vi "Bertta_v09_8.vi"() -> ()   [LabVIEW 2015]
panel:
  out "element":bool
  out "Started:":string
  in  "SHUTDOWN":bool
  in  "MASTER CONTROL":bool
  in  "Tab Control":T1(tab)
  in  "Read Seq":bool
  in  "Save Seq":bool
  in  "Configuration file":path=path "C:/Users/shresplab/Desktop/BerttaConfiguration.lvm" caption="Filename"
  in  "OK Button 2":bool
  out "Boolean":bool
  in  "User (initials)":string
  in  "Project name":string
  in  "Description":string
  out "Output file":string
  out "PUMP1":bool
  out "Target amount":dbl
  out "Scale weight":dbl
  out "Amount now":dbl
  out "Flow rate":dbl
  out "Time to target":dbl format="%<%H:%M:%S>t"
  out "Current step":dbl
  out "Target":dbl
  out "Amount now":dbl
  out "Amount now":dbl
  out "Target":dbl
  out "Current step":dbl
  out "Time to target":dbl format="%<%H:%M:%S>t"
  out "Flow rate":dbl
  out "Amount now":dbl
  out "Scale weight":dbl
  out "Target amount":dbl
  out "PUMP2":bool
  out "Sensor OK 6":bool
  out "Sensor OK 5":bool
  out "Sensor OK 4":bool
  out "Sensor OK 3":bool
  in  "OK Button":bool
  in  "Add comment":string
  out "PUMP3":bool
  out "Target amount":dbl
  out "Scale weight":dbl
  out "Amount now":dbl
  out "Flow rate":dbl
  out "Time to target":dbl format="%<%H:%M:%S>t"
  out "Current step":dbl
  out "Target":dbl
  out "Amount now":dbl
  out "Tr":dbl
  out "Tj in":dbl
  out "Tj out":dbl
  out "T set":dbl
  out "Current step":i32
  out "RPM":dbl
  out "Torque 2":dbl
  out "Waveform Chart 5":dynamicdata(graph)
  out "Waveform Chart 6":dynamicdata(graph)
  out "Waveform Chart 7":dynamicdata(graph)
  in  "Tab Control 2":T2(tab)
  out "Waveform Chart 3":dynamicdata(graph)
  out "Waveform Chart 8":dynamicdata(graph)
  out "Waveform Chart 11":dynamicdata(graph)
  out "Waveform Chart 13":dynamicdata(graph)
  out "Waveform Chart 9":dynamicdata(graph)
  out "Table":string[][](table)=[["14.8.2017 18.06.59", "0,000000", "417,670000", "-0,150000", "1,000000", "22,220000", "23,366837", "23,574959", "23,985852", "23,690000", "240,000000", "4,000000", "0,000000", "397,000000", "-397,000000", "1,000000"], ["14.8.2017 18.07.06", "0,000000", "417,640000", "-0,120000", "1,000000", "22,220000", "23,763115", "23,906257", "23,985694", "23,680000", "240,000000", "4,000000", "0,000000", "397,000000", "-397,000000", "1,000000"], ["14.8.2017 18.07.13", "0,000000", "417,640000", "-0,120000", "1,000000", "22,220000", "23,965922", "24,013440", "23,984906", "23,670000", "240,000000", "4,100000", "3,000000", "397,000000", "-397,000000", "1,000000"], ["14.8.2017 18.07.21", "0,000000", "417,640000", "-0,120000", "1,000000", "22,220000", "23,943860", "23,900110", "23,987113", "23,670000", "240,000000", "4,000000", "0,000000", "397,000000", "-397,000000", "1,000000"], ["14.8.2017 18.07.28", "0,000000", "417,640000", "-0,120000", "1,000000", "22,220000", "23,736328", "23,600018", "23,989004", "23,660000", "240,000000", "4,000000", "0,000000", "397,000000", "-397,000000", "1,000000"], ["14.8.2017 18.07.36", "0,000000", "417,640000", "-0,120000", "1,000000", "22,220000", "23,480910", "23,324538", "23,991053", "23,660000", "240,000000", "4,000000", "0,000000", "397,000000", "-397,000000", "1,000000"], ["14.8.2017 18.07.43", "0,000000", "417,640000", "-0,120000", "2,000000", "22,220000", "23,195579", "23,008270", "23,999093", "23,650000", "240,000000", "4,000000", "0,000000", "397,000000", "-397,000000", "1,000000"], ["14.8.2017 18.07.51", "0,000000", "417,650000", "-417,650000", "1,000000", "22,220000", "22,862541", "22,649021", "24,003979", "23,650000", "240,000000", "4,000000", "0,000000", "397,000000", "-397,000000", "2,000000"], ["14.8.2017 18.07.58", "0,000000", "417,640000", "0,010000", "1,000000", "22,220000", "22,541353", "22,354878", "24,005398", "23,650000", "240,000000", "4,000000", "0,000000", "397,000000", "-397,000000", "1,000000"], ["14.8.2017 18.08.06", "0,000000", "417,640000", "0,010000", "1,000000", "22,220000", "22,347931", "22,253738", "24,007605", "23,640000", "240,000000", "4,100000", "0,000000", "397,000000", "-397,000000", "1,000000"], ["14.8.2017 18.08.13", "0,000000", "417,640000", "0,010000", "1,000000", "22,220000", "22,329030", "22,302102", "24,006028", "23,640000", "240,000000", "4,000000", "0,000000", "395,820000", "-395,820000", "1,000000"], ["14.8.2017 18.08.20", "0,000000", "417,640000", "0,010000", "1,000000", "22,220000", "22,466849", "22,511320", "24,002403", "23,630000", "240,000000", "4,000000", "0,000000", "395,830000", "-0,010000", "1,000000"], ["14.8.2017 18.08.28", "0,000000", "417,640000", "0,010000", "1,000000", "22,220000", "22,707062", "22,835101", "24,000984", "23,620000", "240,000000", "4,000000", "0,000000", "395,830000", "-0,010000", "1,000000"], ["14.8.2017 18.08.35", "0,000000", "417,640000", "0,010000", "1,000000", "22,220000", "23,054104", "23,232979", "24,001299", "23,600000", "240,000000", "4,000000", "0,000000", "395,830000", "-0,010000", "1,000000"], ["14.8.2017 18.08.43", "0,000000", "417,640000", "0,010000", "1,000000", "22,220000", "23,412371", "23,522793", "24,002560", "23,590000", "240,000000", "4,000000", "0,000000", "395,820000", "0,000000", "1,000000"], ["14.8.2017 18.08.51", "0,000000", "417,640000", "0,010000", "1,000000", "22,220000", "23,596247", "23,656125", "24,003821", "23,580000", "240,000000", "4,000000", "0,000000", "395,820000", "0,000000", "1,000000"]]
  in  "Reset":bool
  in  "Temp5":dbl=20.0
  in  "Temp4":dbl=30.0
  in  "Temp3":dbl=40.0
  in  "Temp2":dbl=30.0
  in  "Temp1":dbl=20.0
  out "Boolean 12":bool
  out "Boolean 7":bool
  out "Boolean 6":bool
  out "Boolean 5":bool
  out "Boolean 4":bool
  out "Boolean 19":bool
  in  "Time1":dbl=5.0
  in  "Time2":dbl=5.0
  in  "Time3":dbl=5.0
  in  "Time4":dbl=5.0
  in  "T ext / T ext 2":enum32{"External 1", "External 2"}(radio)
  out "Sensor OK":bool
  in  "T fail":dbl=20.0
  in  "?":bool
  in  "T manual setpoint":dbl=20.0
  in  "Lauda port":dbl=9.0
  in  "Manual select":enum32{"Tr", "Tj"}(radio)
  in  "PAUSE":bool
  out "Waveform Chart":dynamicdata(graph)
  out "T external 2":dbl
  out "Led11 5":bool
  in  "Radio Buttons 4":enum32{"Reglo Digital", "Reglo Analog", "PAM"}(radio)
  out "Speed":dbl
  out "mA":dbl format="%#_2g"
  in  "Port":i32=16
  out "RPM":dbl format="%_4f"
  out "Led10 3":bool
  out "Led9 3":bool
  out "Led8 3":bool
  out "Led7 3":bool
  out "Led6 3":bool
  out "Led5 3":bool
  out "Led4 3":bool
  out "Led3 3":bool
  out "Led2 3":bool
  out "Led1 3":bool
  in  "PumpSeq 4":dbl[][](array[numeric])=[[1.0, 1.0, 0.0, 0.0, 0.0, 0.0, 0.0, 0.0, 0.0, 0.0], [2.0, 1.0, 0.0, 0.0, 0.0, 0.0, 0.0, 0.0, 0.0, 0.0], [3.0, 1.0, 0.0, 0.0, 0.0, 0.0, 0.0, 0.0, 0.0, 0.0], [0.0, 0.0, 0.0, 0.0, 0.0, 0.0, 0.0, 0.0, 0.0, 0.0], [0.0, 0.0, 0.0, 0.0, 0.0, 0.0, 0.0, 0.0, 0.0, 0.0], [0.0, 0.0, 0.0, 0.0, 0.0, 0.0, 0.0, 0.0, 0.0, 0.0], [0.0, 0.0, 0.0, 0.0, 0.0, 0.0, 0.0, 0.0, 0.0, 0.0], [0.0, 0.0, 0.0, 0.0, 0.0, 0.0, 0.0, 0.0, 0.0, 0.0], [0.0, 0.0, 0.0, 0.0, 0.0, 0.0, 0.0, 0.0, 0.0, 0.0], [0.0, 0.0, 0.0, 0.0, 0.0, 0.0, 0.0, 0.0, 0.0, 0.0]]
  in  "?":bool
  out "Flow rate (g/min)":dbl
  out "Scale reading":dbl
  out "Step amount now":dbl
  in  "Grams / min":dbl
  out "Waveform Chart 14":dynamicdata(graph)
  in  "?":bool
  out "Total amount now":dbl
  out "Led11 4":bool
  in  "Reset 5":bool
  out "Elapsed / step":i32
  out "Time to target":dbl format="%<%H:%M:%S>t"
  out "Led11":bool
  in  "Radio Buttons 2":enum32{"Reglo Digital", "Reglo Analog", "PAM"}(radio)
  out "Speed":dbl
  out "mA":dbl format="%#_2g"
  in  "Port":i32=15
  out "RPM":dbl format="%_4f"
  out "Led10":bool
  out "Led9":bool
  out "Led8":bool
  out "Led7":bool
  out "Led6":bool
  out "Led5":bool
  out "Led4":bool
  out "Led3":bool
  out "Led2":bool
  out "Led1":bool
  in  "PumpSeq 2":dbl[][](array[numeric])=[[0.0, 0.0, 0.0, 0.0, 0.0, 0.0, 0.0, 0.0, 0.0, 0.0], [0.0, 0.0, 0.0, 0.0, 0.0, 0.0, 0.0, 0.0, 0.0, 0.0], [0.0, 0.0, 0.0, 0.0, 0.0, 0.0, 0.0, 0.0, 0.0, 0.0], [0.0, 0.0, 0.0, 0.0, 0.0, 0.0, 0.0, 0.0, 0.0, 0.0], [0.0, 0.0, 0.0, 0.0, 0.0, 0.0, 0.0, 0.0, 0.0, 0.0], [0.0, 0.0, 0.0, 0.0, 0.0, 0.0, 0.0, 0.0, 0.0, 0.0], [0.0, 0.0, 0.0, 0.0, 0.0, 0.0, 0.0, 0.0, 0.0, 0.0], [0.0, 0.0, 0.0, 0.0, 0.0, 0.0, 0.0, 0.0, 0.0, 0.0], [0.0, 0.0, 0.0, 0.0, 0.0, 0.0, 0.0, 0.0, 0.0, 0.0], [0.0, 0.0, 0.0, 0.0, 0.0, 0.0, 0.0, 0.0, 0.0, 0.0]]
  in  "?":bool
  out "Flow rate (g/min)":dbl
  out "Scale reading":dbl
  out "Step amount now":dbl
  in  "Grams / min":dbl
  out "Waveform Chart 10":dynamicdata(graph)
  in  "?":bool
  out "Total amount now":dbl
  out "Led11":bool
  in  "Reset 3":bool
  out "Elapsed / step":i32
  out "Time to target":dbl format="%<%H:%M:%S>t"
  out "Led11 3":bool
  in  "Radio Buttons 3":enum32{"Reglo Digital", "Reglo Analog", "PAM"}(radio)
  out "Speed":dbl
  out "mA":dbl format="%#_2g"
  in  "Port":i32=14
  out "RPM":dbl format="%_4f"
  out "Led10 2":bool
  out "Led9 2":bool
  out "Led8 2":bool
  out "Led7 2":bool
  out "Led6 2":bool
  out "Led5 2":bool
  out "Led4 2":bool
  out "Led3 2":bool
  out "Led2 2":bool
  out "Led1 2":bool
  in  "PumpSeq 3":dbl[][](array[numeric])=[[1.0, 3.0, 0.0, 0.0, 0.0, 0.0, 0.0, 0.0, 0.0, 0.0], [2.0, 3.0, 0.0, 0.0, 0.0, 0.0, 0.0, 0.0, 0.0, 0.0], [3.0, 3.0, 0.0, 0.0, 0.0, 0.0, 0.0, 0.0, 0.0, 0.0], [0.0, 0.0, 0.0, 0.0, 0.0, 0.0, 0.0, 0.0, 0.0, 0.0], [0.0, 0.0, 0.0, 0.0, 0.0, 0.0, 0.0, 0.0, 0.0, 0.0], [0.0, 0.0, 0.0, 0.0, 0.0, 0.0, 0.0, 0.0, 0.0, 0.0], [0.0, 0.0, 0.0, 0.0, 0.0, 0.0, 0.0, 0.0, 0.0, 0.0], [0.0, 0.0, 0.0, 0.0, 0.0, 0.0, 0.0, 0.0, 0.0, 0.0], [0.0, 0.0, 0.0, 0.0, 0.0, 0.0, 0.0, 0.0, 0.0, 0.0], [0.0, 0.0, 0.0, 0.0, 0.0, 0.0, 0.0, 0.0, 0.0, 0.0]]
  in  "?":bool
  out "Flow rate (g/min)":dbl
  out "Scale reading":dbl
  out "Step amount now":dbl
  in  "Grams / min":dbl
  out "Waveform Chart 12":dynamicdata(graph)
  in  "?":bool
  out "Total amount now":dbl
  out "Led11 2":bool
  in  "Reset 4":bool
  out "Elapsed / step":i32
  out "Time to target":dbl format="%<%H:%M:%S>t"
  in  "Bypass select 2":enum32{"Remote", "Manual"}(radio)=enum."Manual"
  in  "Port":dbl=13.0
  out "RPM":dbl
  out "Torque":dbl
  in  "Set RPM":dbl(slide) scale=0.0..2000.0
  out "Waveform Chart 4":dynamicdata(graph)
  in  "Treshold (T/C)":dbl=0.5
  out "DAQ 9217 (PT100)":errorcluster
  out "Config File":dbl[][](array[numeric])
  # "Temperature sensor:"
  # "Manual control:"
  # "PUMP & SCALE 1"
  # "STEP"
  # "TOTAL"
  # "PUMP & SCALE 2"
  # "STEP"
  # "TOTAL"
  # "PUMP & SCALE 3"
  # "STEP"
  # "TOTAL"
  # "Manual control"
  # "Secondary temperature sensor"
  # "Device communication"
  # "Temp"
  # "Time"
  # "Grams    /   min"
  # "End of sequence"
  # "Manual control"
  # "Device communication"
  # "Pump configuration"
  # "Grams    /   min"
  # "End of sequence"
  # "Manual control"
  # "Device communication"
  # "Pump configuration"
  # "Grams    /   min"
  # "End of sequence"
  # "Manual control"
  # "Device communication"
  # "Pump configuration"
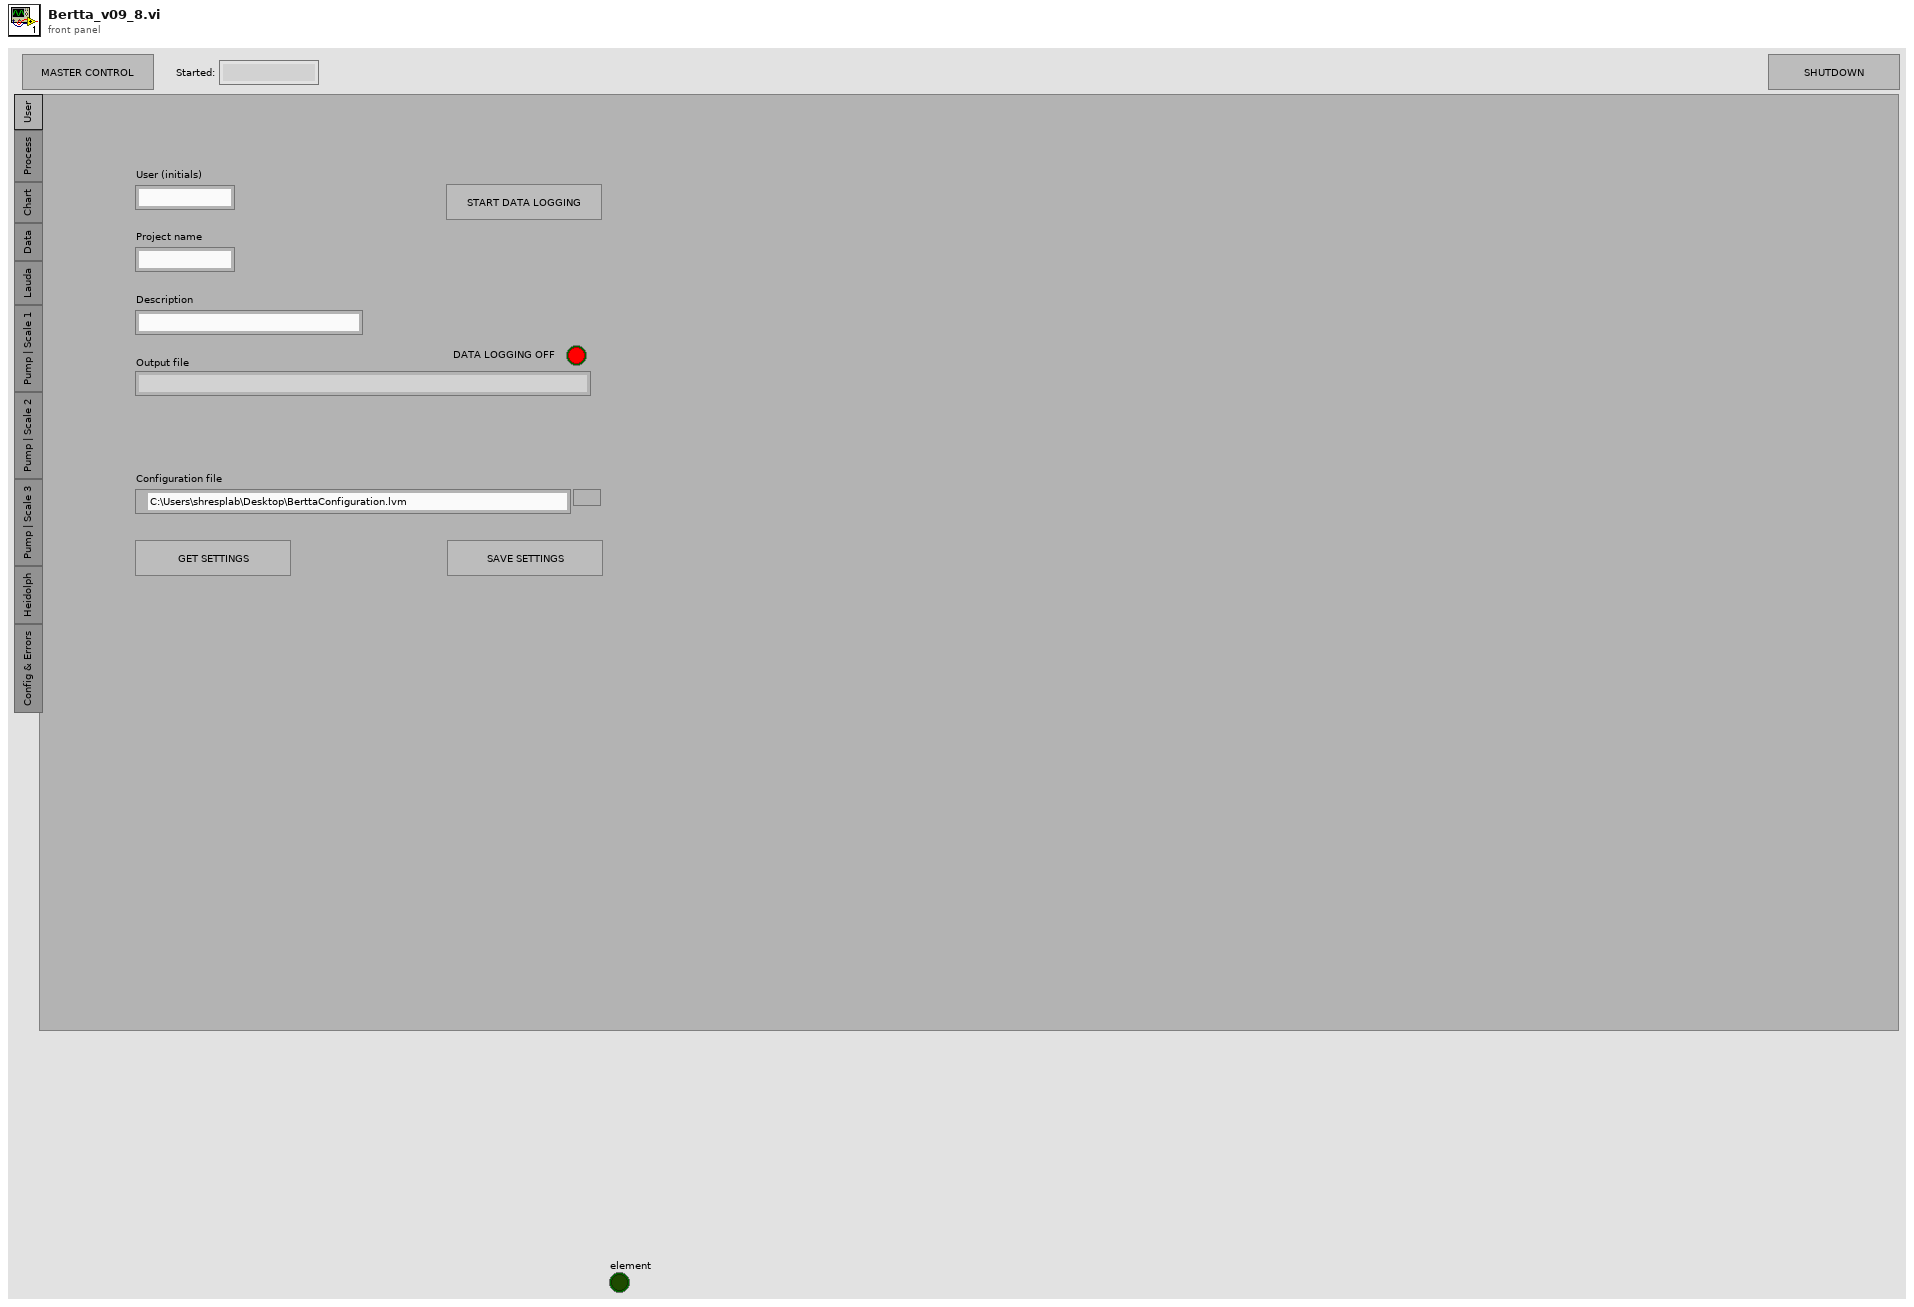
[diagram p1: front panel]
types:
  T1 = enum32{"User", "Process", "Chart", "Data", "Lauda", "Pump | Scale 1", "Pump | Scale 2", "Pump | Scale 3", "Heidolph", "Config & Errors"}
  T2 = enum32{"Temperatures", "Scale / Pump 1", "Scale / Pump 2", "Scale / Pump 3", "RPM / torque"}
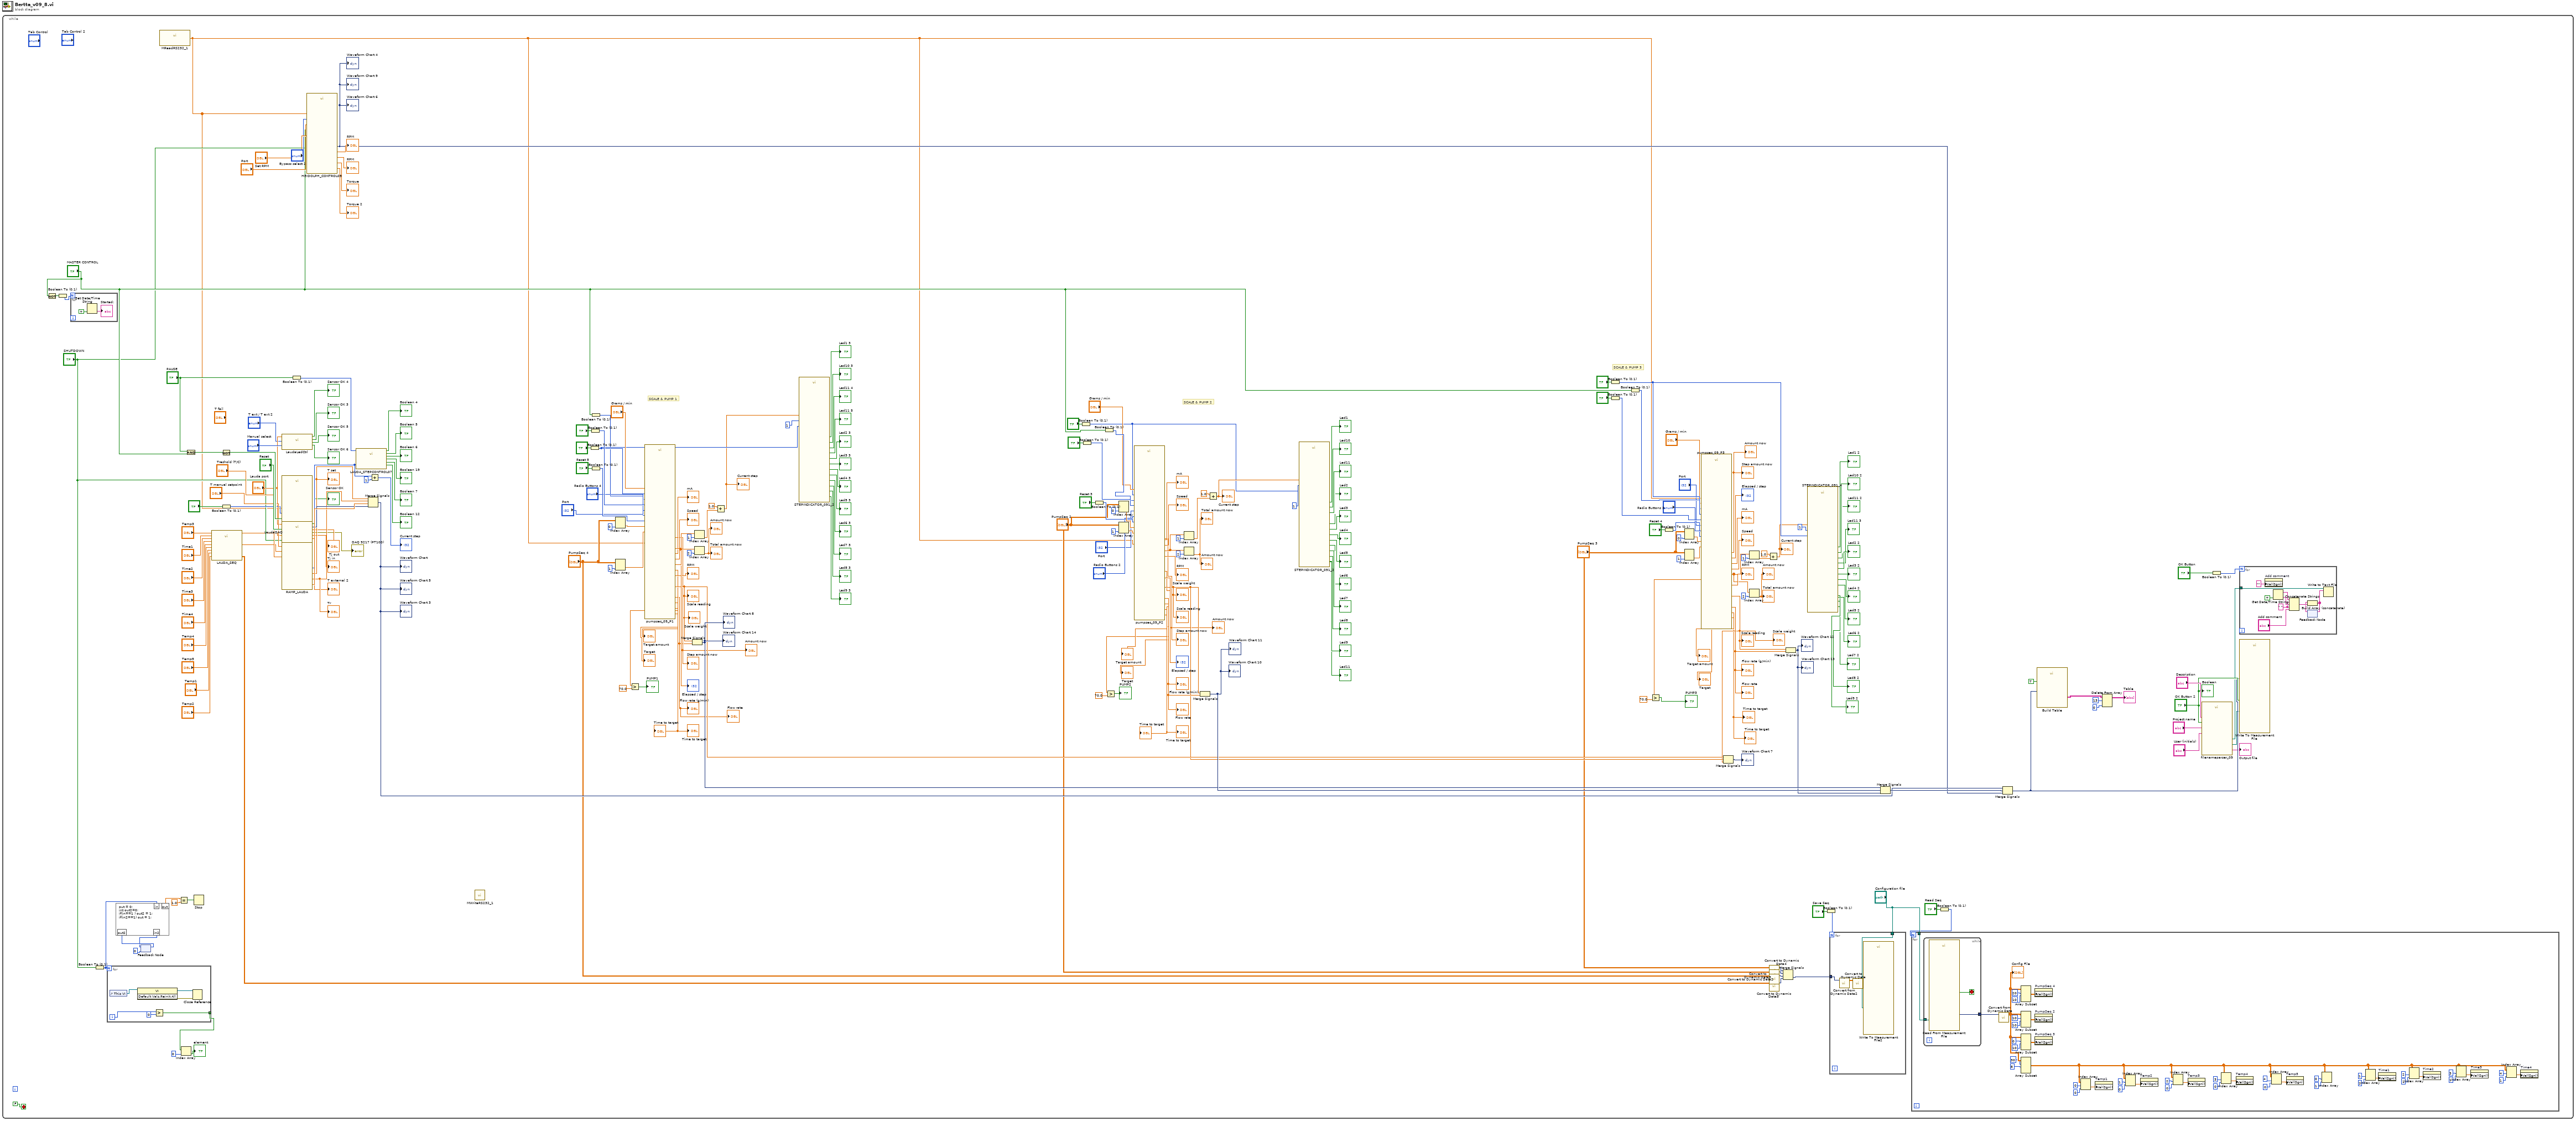
[diagram p0: block diagram]
diagram:
  n1 = while {
    stop <- FALSE stop-if-true
    # "SCALE & PUMP 1"
    # "SCALE & PUMP 3"
    # "SCALE & PUMP 2"
    n2 = Not(x="MASTER CONTROL") -> (.not. x?=w228:bool)
    n3 = Boolean To (0,1)(Boolean=w228) -> (0, 1=w229:i16)
    n4 = for {
      N: w229 -> [_]
      n5 = Get Date/Time String(want seconds? (F)=TRUE) -> (time string=→"Started:":string)  [unwired: 2 in, 1 out]
    }
    n6 = Boolean To (0,1)(Boolean="SHUTDOWN") -> (0, 1=w210:i16)
    n7 = for {
      N: w210 -> [_]
      tunnel: [w307] -> w227 mode=indexing
      i -> [w309]
      n8 = control-ref of="This VI"() -> (w312:refnum<vi>)
      n9 = invoke class="VI" method="Default Vals.Reinit All"(reference=w312) -> (reference out=w310:refnum<vi>, error out=w311:errorcluster)  [unwired: 2 in, 1 out]
      n10 = Greater?(x=w309, y=0) -> (0:w307:bool)
      n11 = Close Reference(reference=w310, error in (no error)=w311) -> ()  [unwired: 1 out]
    }
    n12 = feedback #1(0) -> (w208:i32)
    n13 = formula code="out = 0;\nint out2=0;\nif(in==1 ) out2 = 1;\nif(in2==1) out = 1;"("in"=w210, "in2"=w208) -> ("out"=w212:dbl, "out2"=w209:i32)
    n14 = feedback-in #1(w209) -> ()
    n15 = call "MReadRS232_1.vi"() -> ("params"=w1:dbl[])  [unwired: 11 in]
    n16 = Equal?(x=w212, y=1.0) -> (x = y?=w211:bool)
    n17 = Index Array(array=w227, index=0) -> (element=→"element":bool)
    n18 = And(x="PAUSE", y="MASTER CONTROL") -> (x .and. y?=w166:bool)
    n19 = Stop(stop? (T)=w211) -> ()
    n20 = call "LAUDA_SEQ.vi"("Numeric 2"="Temp3", "Numeric 1"="Temp2", "Numeric"="Temp1", "Numeric 5"="Time1", "Numeric 6"="Time2", "Numeric 7"="Time3", "Numeric 8"="Time4", "Numeric 3"="Temp4", "Numeric 4"="Temp5") -> ("output array"=w8:dbl[], "output array 2"=w9:dbl[], "appended array"=w7:dbl[][])  [unwired: 4 in]
    n21 = Not(x=w166) -> (.not. x?=w165:bool)
    n22 = Boolean To (0,1)(Boolean="?") -> (0, 1=w153:i16)
    n23 = call "LaudaLedCtrl.vi"("Manual select"="Manual select", "T ext / T ext in"="T ext / T ext 2", "Lauda port"="Lauda port") -> ("Sensor OK 5"=→"Sensor OK 5":bool, "Sensor OK 3"=→"Sensor OK 3":bool, "Sensor OK 4"=→"Sensor OK 4":bool, "Sensor OK 6"=→"Sensor OK 6":bool)  [unwired: 5 in]
    n24 = call "RAMP_LAUDA.vi"("pause"=w165, "manual"=w153, "Array"=w1, "T_man"="T manual setpoint", "Seq"=w8, "reset"="Reset", "TimeParams"=w9, "shutdown"="SHUTDOWN", "port"="Lauda port", "treshold"="Treshold (T/C)") -> ("T in"=w64:dbl, "STEP"=w32:i32, "T ext"=w50:dbl, "T control"=w51:dbl)  [unwired: 1 in, 1 out]
    "Tr" <- w50
    "T set" <- w51
    n25 = call "LaudaDAQ.vi"() -> ("error out"=→"DAQ 9217 (PT100)":errorcluster, 1:"Tj out"=→"Tj out":dbl, "data"=w63:dynamicdata, "Sensor OK"=→"Sensor OK":bool, 4:"Tj out"=→"Tj in":dbl, "T external 2"=→"T external 2":dbl)  [unwired: 6 in]
    n26 = Boolean To (0,1)(Boolean="PAUSE") -> (0, 1=w205:i16)
    n27 = call "HEIDOLPH_CONTROL09.vi"("master"="MASTER CONTROL", "Array"=w1, "shutdown"="SHUTDOWN", "Bypass select"="Bypass select 2", "Set RPM"="Set RPM", "Device port"="Port") -> ("Dynamic Data"=w65:dynamicdata, "RPM"=→"RPM":dbl, "RPM 2"=→"RPM":dbl, "Torque"=→"Torque":dbl, "Torque 2"=→"Torque 2":dbl)  [unwired: 1 in]
    "Waveform Chart 4" <- w65
    "Waveform Chart 6" <- w65
    "Waveform Chart 9" <- w65
    n28 = call "LAUDA_STEPCONTROL07.vi"("step"=w32, "pause"=w205) -> ("Boolean 13"=→"Boolean 19":bool, "Boolean 6"=→"Boolean 6":bool, "Boolean 5"=→"Boolean 5":bool, "Boolean 4"=→"Boolean 4":bool, "Boolean 7"=→"Boolean 7":bool, "Boolean 12"=→"Boolean 12":bool)  [unwired: 4 in]
    n29 = Merge Signals(w51, w50, w64, w63) -> (w66:dynamicdata)
    "Waveform Chart 3" <- w66
    "Waveform Chart" <- w66
    "Waveform Chart 5" <- w66
    n30 = Add(x=w32, y=1) -> (x+y=→"Current step":i32)
    n31 = call "MWriteRS232_1.vi"() -> ()  [unwired: 12 in]
    n32 = Boolean To (0,1)(Boolean="?") -> (0, 1=w75:i16)
    n33 = Boolean To (0,1)(Boolean="?") -> (0, 1=w84:i16)
    n34 = Boolean To (0,1)(Boolean="MASTER CONTROL") -> (0, 1=w71:i16)
    n35 = Boolean To (0,1)(Boolean="Reset 5") -> (0, 1=w83:i16)
    n36 = Index Array(array="PumpSeq 4", index (col)=0) -> (element=w88:dbl[])  [unwired: 1 in]
    n37 = Index Array(array="PumpSeq 4", index (col)=1) -> (element=w109:dbl[])  [unwired: 1 in]
    n38 = call "pumpsec_09_P1.vi"("reset"=w83, "master"=w71, "manual"=w75, "pause"=w84, "pump_type"="Radio Buttons 4", "port, Reglo D"="Port", "Array"=w1, "Target"=w88, "fr_manual"="Grams / min", "Time"=w109) -> ("pumpCtrl"=w45:dbl, "totaltarget"=→"Target":dbl, "target_step"=→"Target amount":dbl, "time_to_target"=→"Time to target" →"Time to target":dbl, "step_fr"=w18:dbl, "amount_step"=→"Amount now" →"Step amount now":dbl, "Reglo D"=→"RPM":dbl, "Scale"=w59:dbl, "mA"=→"mA":dbl, "elapsed_step"=→"Elapsed / step":dbl, "params"=w106:dbl[], "PAM"=→"Speed":dbl)  [unwired: 4 in, 2 out]
    "Flow rate" <- w18
    "Scale weight" <- w59
    "Scale reading" <- w59
    "Flow rate (g/min)" <- w18
    n39 = Greater?(x=w45, y=70.0) -> (0:→"PUMP1":bool)
    n40 = Merge Signals(w59, w18) -> (w69:dynamicdata)
    "Waveform Chart 8" <- w69
    "Waveform Chart 14" <- w69
    n41 = Index Array(array=w106, index=1) -> (element=w103:dbl)
    n42 = Index Array(array=w106, index=2) -> (element=→"Amount now" →"Total amount now":dbl)
    n43 = Add(x=1.0, y=w103) -> (x+y=w19:dbl)
    "Current step" <- w19
    n44 = call "STEPINDICATOR_091_2.vi"("current step"=w19, "enable"=i16 1, "manual"=w75) -> ("Led 8"=→"Led8 3":bool, "Led 10"=→"Led10 3":bool, "Led 11"=→"Led11 4":bool, "Led 7"=→"Led7 3":bool, "Led 1"=→"Led1 3":bool, "Led 6"=→"Led6 3":bool, "Led 2"=→"Led2 3":bool, "Led 12"=→"Led11 5":bool, "Led 5"=→"Led5 3":bool, "Led 4"=→"Led4 3":bool, "Led 3"=→"Led3 3":bool, "Led 9"=→"Led9 3":bool)  [unwired: 1 in]
    n45 = Boolean To (0,1)(Boolean="?") -> (0, 1=w148:i16)
    n46 = Boolean To (0,1)(Boolean="?") -> (0, 1=w198:i16)
    n47 = Boolean To (0,1)(Boolean="Reset 3") -> (0, 1=w196:i16)
    n48 = Boolean To (0,1)(Boolean="MASTER CONTROL") -> (0, 1=w190:i16)
    n49 = Index Array(array="PumpSeq 2", index (col)=0 ("disabled index (col)")) -> (element=w201:dbl[])  [unwired: 1 in]
    n50 = Index Array(array="PumpSeq 2", index (col)=1 ("disabled index (col)")) -> (element=w200:dbl[])  [unwired: 1 in]
    n51 = call "pumpsec_09_P2.vi"("reset"=w196, "master"=w190, "manual"=w148, "pause"=w198, "pump_type"="Radio Buttons 2", "port, Reglo D"="Port", "Array"=w1, "Target"=w201, "fr_manual"="Grams / min", "Time"=w200) -> ("pumpCtrl"=w41:dbl, "totaltarget"=→"Target":dbl, "target_step"=→"Target amount":dbl, "time_to_target"=→"Time to target" →"Time to target":dbl, "step_fr"=w62:dbl, "amount_step"=→"Amount now" →"Step amount now":dbl, "Reglo D"=→"RPM":dbl, "Scale"=w58:dbl, "mA"=→"mA":dbl, "elapsed_step"=→"Elapsed / step":dbl, "params"=w191:dbl[], "PAM"=→"Speed":dbl)  [unwired: 4 in, 2 out]
    "Scale weight" <- w58
    "Flow rate" <- w62
    "Scale reading" <- w58
    "Flow rate (g/min)" <- w62
    n52 = Greater?(x=w41, y=70.0) -> (0:→"PUMP2":bool)
    n53 = Index Array(array=w191, index=1) -> (element=w194:dbl)
    n54 = Index Array(array=w191, index=2) -> (element=→"Amount now" →"Total amount now":dbl)
    n55 = Merge Signals(w58, w62) -> (w72:dynamicdata)
    "Waveform Chart 11" <- w72
    "Waveform Chart 10" <- w72
    n56 = Add(x=1.0, y=w194) -> (x+y=w184:dbl)
    "Current step" <- w184
    n57 = call "STEPINDICATOR_091_2.vi"("current step"=w184, "enable"=i16 1, "manual"=w148) -> ("Led 8"=→"Led8":bool, "Led 10"=→"Led10":bool, "Led 11"=→"Led11":bool, "Led 7"=→"Led7":bool, "Led 1"=→"Led1":bool, "Led 6"=→"Led6":bool, "Led 2"=→"Led2":bool, "Led 12"=→"Led11":bool, "Led 5"=→"Led5":bool, "Led 4"=→"Led4":bool, "Led 3"=→"Led3":bool, "Led 9"=→"Led9":bool)  [unwired: 1 in]
    n58 = Boolean To (0,1)(Boolean="?") -> (0, 1=w142:i16)
    n59 = Boolean To (0,1)(Boolean="?") -> (0, 1=w141:i16)
    n60 = Boolean To (0,1)(Boolean="MASTER CONTROL") -> (0, 1=w143:i16)
    n61 = Boolean To (0,1)(Boolean="Reset 4") -> (0, 1=w122:i16)
    n62 = Index Array(array="PumpSeq 3", index (col)=0 ("disabled index (col)")) -> (element=w125:dbl[])  [unwired: 1 in]
    n63 = Index Array(array="PumpSeq 3", index (col)=1 ("disabled index (col)")) -> (element=w124:dbl[])  [unwired: 1 in]
    n64 = call "pumpsec_09_P3.vi"("reset"=w122, "master"=w143, "manual"=w142, "pause"=w141, "pump_type"="Radio Buttons 3", "port, Reglo D"="Port", "Array"=w1, "Target"=w125, "fr_manual"="Grams / min", "Time"=w124) -> ("pumpCtrl"=w38:dbl, "totaltarget"=→"Target":dbl, "target_step"=→"Target amount":dbl, "time_to_target"=→"Time to target" →"Time to target":dbl, "step_fr"=w61:dbl, "amount_step"=→"Amount now" →"Step amount now":dbl, "Reglo D"=→"RPM":dbl, "Scale"=w57:dbl, "mA"=→"mA":dbl, "elapsed_step"=→"Elapsed / step":dbl, "params"=w111:dbl[], "PAM"=→"Speed":dbl)  [unwired: 4 in, 2 out]
    "Scale weight" <- w57
    "Flow rate" <- w61
    "Scale reading" <- w57
    "Flow rate (g/min)" <- w61
    n65 = Greater?(x=w38, y=70.0) -> (0:→"PUMP3":bool)
    n66 = Merge Signals(w59, w58, w57) -> (→"Waveform Chart 7":dynamicdata)
    n67 = Index Array(array=w111, index=1) -> (element=w112:dbl)
    n68 = Index Array(array=w111, index=2) -> (element=→"Amount now" →"Total amount now":dbl)
    n69 = Add(x=1.0, y=w112) -> (x+y=w110:dbl)
    "Current step" <- w110
    n70 = call "Convert to Dynamic Data4"("2D Array"="PumpSeq 3") -> ("Dynamic Data Type"=w10:dynamicdata)  [unwired: 3 in]
    n71 = call "Convert to Dynamic Data3"("2D Array"="PumpSeq 2") -> ("Dynamic Data Type"=w12:dynamicdata)  [unwired: 3 in]
    n72 = call "Convert to Dynamic Data2"("2D Array"="PumpSeq 4") -> ("Dynamic Data Type"=w15:dynamicdata)  [unwired: 3 in]
    n73 = call "Convert to Dynamic Data5"("2D Array"=w7) -> ("Dynamic Data Type"=w6:dynamicdata)  [unwired: 3 in]
    n74 = Merge Signals(w10, w12, w15, w6) -> (w14:dynamicdata)
    n75 = Merge Signals(w57, w61) -> (w68:dynamicdata)
    "Waveform Chart 13" <- w68
    "Waveform Chart 12" <- w68
    n76 = call "STEPINDICATOR_091_4.vi"("current step"=w110, "enable"=i16 1, "manual"=w142) -> ("Led 8"=→"Led8 2":bool, "Led 10"=→"Led10 2":bool, "Led 11"=→"Led11 2":bool, "Led 7"=→"Led7 2":bool, "Led 1"=→"Led1 2":bool, "Led 6"=→"Led6 2":bool, "Led 2"=→"Led2 2":bool, "Led 12"=→"Led11 3":bool, "Led 5"=→"Led5 2":bool, "Led 4"=→"Led4 2":bool, "Led 3"=→"Led3 2":bool, "Led 9"=→"Led9 2":bool)  [unwired: 1 in]
    n77 = Boolean To (0,1)(Boolean="Save Seq") -> (0, 1=w4:i16)
    n78 = for {
      N: w4 -> [_]
      tunnel: w14 -> [w304]
      tunnel: "Configuration file" -> [w305]
      n79 = call "Convert from Dynamic Data2"("Dynamic Data Type"=w304) -> ("Array"=w303:dbl[][])  [unwired: 3 in]
      n80 = call "Convert to Dynamic Data"("2D Array"=w303) -> ("Dynamic Data Type"=w306:dynamicdata)  [unwired: 3 in]
      n81 = call "Write To Measurement File2"("Signals"=w306, "Filename"=w305) -> ()  [unwired: 15 in, 3 out]
    }
    n82 = Merge Signals(w69, w72, w68) -> (w67:dynamicdata)
    n83 = Boolean To (0,1)(Boolean="Read Seq") -> (0, 1=w2:i16)
    n84 = for {
      N: w2 -> [_]
      tunnel: "Configuration file" -> [w256]
      n85 = while {
        tunnel: [w302] -> w299
        tunnel: w256 -> [w301]
        stop <- w300 stop-if-true
        n86 = call "Read From Measurement File"("Filename"=w301) -> ("Signals"=w302:dynamicdata, "EOF?"=w300:bool)  [unwired: 5 in, 4 out]
      }
      n87 = call "Convert from Dynamic Data"("Dynamic Data Type"=w299) -> ("Array"=w289:dbl[][])  [unwired: 3 in]
      "Config File" <- w289
      n88 = Array Subset(array=w289, index (row)=20 ("index"), length (row)=10 ("length")) -> (w296:dbl[][])  [unwired: 2 in]
      n89 = Array Subset(array=w289, index (row)=10 ("index"), length (row)=10 ("length")) -> (w291:dbl[][])  [unwired: 2 in]
      n90 = Array Subset(array=w289, index (row)=0 ("index"), length (row)=10 ("length")) -> (w290:dbl[][])  [unwired: 2 in]
      n91 = Array Subset(array=w289, index (row)=30 ("index"), length (row)=8 ("length")) -> (w266:dbl[][])  [unwired: 2 in]
      n92 = property on="PumpSeq 4" class="Arr (strict)"("Val(Sgnl)"=w296) -> ()  [unwired: 2 in, 2 out]
      n93 = property on="PumpSeq 2" class="Arr (strict)"("Val(Sgnl)"=w291) -> ()  [unwired: 2 in, 2 out]
      n94 = property on="PumpSeq 3" class="Arr (strict)"("Val(Sgnl)"=w290) -> ()  [unwired: 2 in, 2 out]
      n95 = Index Array(array=w266, index (row)=0, index (col)=0 ("disabled index (col)")) -> (element=w265:dbl)
      n96 = property on="Temp1" class="DigNum (strict)"("Val(Sgnl)"=w265) -> ()  [unwired: 2 in, 2 out]
      n97 = Index Array(array=w266, index (row)=1, index (col)=0 ("disabled index (col)")) -> (element=w264:dbl)
      n98 = property on="Temp2" class="DigNum (strict)"("Val(Sgnl)"=w264) -> ()  [unwired: 2 in, 2 out]
      n99 = Index Array(array=w266, index (row)=2, index (col)=0 ("disabled index (col)")) -> (element=w263:dbl)
      n100 = property on="Temp3" class="DigNum (strict)"("Val(Sgnl)"=w263) -> ()  [unwired: 2 in, 2 out]
      n101 = Index Array(array=w266, index (row)=3, index (col)=0 ("disabled index (col)")) -> (element=w262:dbl)
      n102 = property on="Temp4" class="DigNum (strict)"("Val(Sgnl)"=w262) -> ()  [unwired: 2 in, 2 out]
      n103 = Index Array(array=w266, index (row)=4, index (col)=0 ("disabled index (col)")) -> (element=w261:dbl)
      n104 = property on="Temp5" class="DigNum (strict)"("Val(Sgnl)"=w261) -> ()  [unwired: 2 in, 2 out]
      n105 = Index Array(array=w266, index (row)=0, index (col)=1 ("disabled index (col)")) -> ()  [unwired: 1 out]
      n106 = Index Array(array=w266, index (row)=1, index (col)=1 ("disabled index (col)")) -> (element=w260:dbl)
      n107 = property on="Time1" class="DigNum (strict)"("Val(Sgnl)"=w260) -> ()  [unwired: 2 in, 2 out]
      n108 = Index Array(array=w266, index (row)=2, index (col)=1 ("disabled index (col)")) -> (element=w259:dbl)
      n109 = property on="Time2" class="DigNum (strict)"("Val(Sgnl)"=w259) -> ()  [unwired: 2 in, 2 out]
      n110 = Index Array(array=w266, index (row)=3, index (col)=1 ("disabled index (col)")) -> (element=w258:dbl)
      n111 = property on="Time3" class="DigNum (strict)"("Val(Sgnl)"=w258) -> ()  [unwired: 2 in, 2 out]
      n112 = Index Array(array=w266, index (row)=4, index (col)=1 ("disabled index (col)")) -> (element=w257:dbl)
      n113 = property on="Time4" class="DigNum (strict)"("Val(Sgnl)"=w257) -> ()  [unwired: 2 in, 2 out]
    }
    n114 = Merge Signals(w66, w67, w65) -> (w222:dynamicdata)
    n115 = call "Build Table"("Include time data"=TRUE, "Signals"=w222) -> ("Table"=w221:string[][])  [unwired: 3 in, 6 out]
    n116 = Delete From Array(array=w221, length=13, index (col)=0 ("index (row)")) -> (array with subset deleted=→"Table":string[][])  [unwired: 1 in, 1 out]
    n117 = call "filenameparser_09.vi"("Description"="Description", "Project name"="Project name", "User (initials)"="User (initials)", "OK Button in"="OK Button 2") -> ("Output file"=→"Output file":string, "appended path 2"=w217:path, "appended path"=w216:path)  [unwired: 5 in]
    n118 = Boolean To (0,1)(Boolean="OK Button") -> (0, 1=w215:i16)
    n119 = for {
      N: w215 -> [_]
      tunnel: w216 -> [w248]
      w252 = " " ("string")
      n120 = property on="Add comment" class="Str"("Val(Sgnl)"="" ("Value (Signaling)")) -> ()  [unwired: 2 in, 2 out]
      n121 = Get Date/Time String(want seconds? (F)=TRUE) -> (date string=w255:string, time string=w253:string)  [unwired: 2 in]
      n122 = Concatenate Strings(w255, w252, w253, w252, "Add comment") -> (w251:string)
      n123 = feedback #2() -> (w250:string[])  [unwired: 1 in]
      n124 = Build Array (concatenate)(w250, w251) -> (w249:string[])
      n125 = feedback-in #2(w249) -> ()
      n126 = Write to Text File(file (use dialog)=w248, text=w249) -> ()  [unwired: 2 in, 3 out]
    }
    n127 = call "Write To Measurement File"("Signals"=w222, "Enable"="OK Button 2", "Filename"=w217) -> ()  [unwired: 14 in, 3 out]
    "Boolean" <- "OK Button 2"
  }
